vi "CSEI.vi"() -> ()   [LabVIEW 2010]
uses:
  <vilib>/addons/Simulation Interface/_sitctls/sit Indicator Info.ctl
  <vilib>/addons/Simulation Interface/_sitctls/sit Indicator Type.ctl
  <vilib>/addons/Simulation Interface/_sitctls/sit Client Meta Info (v3).ctl
  <vilib>/addons/Simulation Interface/_sitctls/sit MDL Line Item Info.ctl
  <vilib>/addons/Simulation Interface/_sitctls/sit MDL Line Type.ctl
  <vilib>/addons/Simulation Interface/_sitctls/sit Details Settings.ctl
  <vilib>/addons/Simulation Interface/_sitctls/sit Execution Host.ctl
  <vilib>/addons/Simulation Interface/_sitctls/SIT Sim State.ctl
  <vilib>/Utility/inputDevices.llb/closeJoystick.vi
  <vilib>/Utility/inputDevices.llb/joystickAcquire.vi
  <vilib>/addons/Simulation Interface/_sitclient.llb/NI_SIT_sitclient.lvlib
  <vilib>/addons/Simulation Interface/_sitctls/NI_SIT_sitctls.lvlib
  <vilib>/ptbypt/NI_PtbyPt.lvlib
  <vilib>/picture/3D Picture Control/NI_3D Picture Control.lvlib
panel:
  in  "Reset dp":dbl
  in  "eulerselector":dbl=1.0 min=1.0 max=3.0 step=1.0
  in  "xyz selector":dbl=1.0 min=1.0 max=3.0 step=1.0
  out "SIT1 9":dbl
  out "SIT1 8":dbl
  out "SIT1 7":dbl
  out "SIT1 6":dbl
  out "SIT1 5":dbl
  out "SIT1 4":dbl
  out "SIT1 3":dbl
  out "SIT1 2":dbl
  out "SIT1":dbl
  out "stbd vsp r":dbl
  out "port vsp r":dbl
  in  "DPinputFrom":enum32{"OK Button 4", "OK Button 5"}(radio)
  out "SIT_Status":string
  in  "SIT_stopVI":bool
  in  "SIT_Run":bool
  in  "SIT_Pause":bool
  in  "SIT_Stop":bool
  in  "SIT_Details":bool
  in  "SIT_Remap":bool
  in  "SIT_RVE":bool
  in  "CSE1onoff":bool
  in  "Tab Control":T1(tab)
  out "Main battery half voltage":dbl
  out "Servo Battery":dbl(knob) scale=0.0..8.0
  in  "Left Y":dbl(slide) scale=-32676.0..32676.0
  in  "Left X":dbl(slide) scale=-32676.0..32676.0
  out "Bowthruster Battery":dbl(knob) scale=0.0..8.0
  in  "VSP Speeds":dbl(slide) min=-1.0 max=1.0 step=0.05 scale=-1.0..1.0
  out "Main Battery":dbl(knob) scale=0.0..18.0
  in  "Right Y":dbl(slide) scale=-32676.0..32676.0
  in  "Right X":dbl(slide) scale=-32676.0..32676.0
  in  "Power Limiter":dbl(slide) min=0.0 max=1.0 step=0.05 scale=0.0..1.0
  out "Direction L VSP":dbl(knob) scale=180.0..-180.0
  out "Direction R VSP":dbl(knob) scale=180.0..-180.0
  out "Magnitude Pitch L VSP":dbl(knob) scale=0.0..1.0
  out "Magnitude Pitch R VSP":dbl(knob) scale=0.0..1.0
  out "Slide BT green":dbl(slide) scale=0.0..1.0
  out "Slide BT red":dbl(slide)
  out "X button":bool
  out "square":bool
  out "triangle":bool
  out "circle":bool
  out "leftJoystick":bool
  out "rightJoystick":bool
  out "R2button":bool
  out "Dright":bool
  out "Dup":bool
  out "Dleft":bool
  out "Ddown":bool
  out "L2 button":bool
  in  "Eta_d LPF":bool
  in  "Resed DP Int.":bool
  in  "USE cse1 setpoint":bool
  in  "Show HIL":bool
  in  "Show CSEI":bool
  in  "Wave Filter":bool
  in  "K_d":dbl(slide) min=0.0 max=5.0 step=0.25 scale=0.0..5.0
  in  "K_i":dbl(slide) min=0.0 max=5.0 step=0.25 scale=0.0..5.0
  in  "K_p":dbl(slide) min=0.0 max=10.0 step=0.5 scale=0.0..10.0
  out "Vis Yaw":dbl
  out "Vis Pitch":dbl
  out "Vis Roll":dbl
  out "Vis Z":dbl
  out "Vis Y":dbl
  out "Vis X":dbl
  in  "OK Button":bool
  in  "Reset States":dbl
  in  "HIL -> CSE1":bool
  in  "eta_d_Psi":dbl
  in  "eta_d_E":dbl
  in  "eta_d_N":dbl
  out "u5":dbl
  out "u4":dbl
  out "u3":dbl
  out "u2":dbl
  out "u1":dbl
  out "Tau_6":dbl
  out "Tau_2":dbl
  out "Tau_1":dbl
  out "Vis Psi":dbl
  out "Vis E":dbl
  out "Vis N":dbl
  out "3D Picture":refnum<vi>(3d-picture)
  out "Regulation Error Yaw":waveform(dbl)[](graph)
  out "Regulation Error East":waveform(dbl)[](graph)
  out "Regulation Error North":waveform(dbl)[](graph)
  in  "MODE":T2(radio)
  out "Numeric 2":dbl
  out "Numeric":dbl
  in  "Boolean 2":bool
  in  "R2":i32
  in  "L2":i32
  in  "Boolean":bool
  out "Y-axis":i32
  out "X-axis":i32
  out "Joystick Info":T3(array[cluster])
  in  "SIT_Meta_Info":T4
  in  "SIT_Indicator_Indices":T9[](array[typedef])=[{"Indicator Index"=-1, "Number of Signals"=0, "Indicator Type"=enum."Knob"}, {"Indicator Index"=-1, "Number of Signals"=0, "Indicator Type"=enum."Knob"}, {"Indicator Index"=-1, "Number of Signals"=0, "Indicator Type"=enum."Knob"}, {"Indicator Index"=-1, "Number of Signals"=0, "Indicator Type"=enum."Knob"}, {"Indicator Index"=-1, "Number of Signals"=0, "Indicator Type"=enum."Knob"}, {"Indicator Index"=-1, "Number of Signals"=0, "Indicator Type"=enum."Knob"}, {"Indicator Index"=-1, "Number of Signals"=0, "Indicator Type"=enum."Digital"}, {"Indicator Index"=-1, "Number of Signals"=0, "Indicator Type"=enum."Digital"}, {"Indicator Index"=-1, "Number of Signals"=0, "Indicator Type"=enum."Digital"}, {"Indicator Index"=-1, "Number of Signals"=0, "Indicator Type"=enum."WaveformChart"}, {"Indicator Index"=-1, "Number of Signals"=0, "Indicator Type"=enum."WaveformChart"}, {"Indicator Index"=-1, "Number of Signals"=0, "Indicator Type"=enum."WaveformChart"}, {"Indicator Index"=-1, "Number of Signals"=0, "Indicator Type"=enum."Digital"}, {"Indicator Index"=-1, "Number of Signals"=0, "Indicator Type"=enum."Digital"}, {"Indicator Index"=-1, "Number of Signals"=0, "Indicator Type"=enum."Digital"}, {"Indicator Index"=-1, "Number of Signals"=0, "Indicator Type"=enum."Digital"}, {"Indicator Index"=-1, "Number of Signals"=0, "Indicator Type"=enum."Digital"}, {"Indicator Index"=-1, "Number of Signals"=0, "Indicator Type"=enum."Digital"}, {"Indicator Index"=-1, "Number of Signals"=0, "Indicator Type"=enum."Digital"}, {"Indicator Index"=-1, "Number of Signals"=0, "Indicator Type"=enum."Digital"}, {"Indicator Index"=-1, "Number of Signals"=0, "Indicator Type"=enum."Digital"}, {"Indicator Index"=-1, "Number of Signals"=0, "Indicator Type"=enum."Knob"}, {"Indicator Index"=-1, "Number of Signals"=0, "Indicator Type"=enum."Slide"}, {"Indicator Index"=-1, "Number of Signals"=0, "Indicator Type"=enum."Slide"}, {"Indicator Index"=-1, "Number of Signals"=0, "Indicator Type"=enum."Digital"}, {"Indicator Index"=-1, "Number of Signals"=0, "Indicator Type"=enum."Digital"}, {"Indicator Index"=-1, "Number of Signals"=0, "Indicator Type"=enum."Digital"}, {"Indicator Index"=27, "Number of Signals"=1, "Indicator Type"=enum."Digital"}, {"Indicator Index"=28, "Number of Signals"=1, "Indicator Type"=enum."Digital"}, {"Indicator Index"=-1, "Number of Signals"=0, "Indicator Type"=enum."Digital"}, {"Indicator Index"=30, "Number of Signals"=1, "Indicator Type"=enum."Digital"}, {"Indicator Index"=-1, "Number of Signals"=0, "Indicator Type"=enum."Digital"}, {"Indicator Index"=-1, "Number of Signals"=0, "Indicator Type"=enum."Digital"}, {"Indicator Index"=-1, "Number of Signals"=0, "Indicator Type"=enum."Digital"}, {"Indicator Index"=-1, "Number of Signals"=0, "Indicator Type"=enum."Digital"}, {"Indicator Index"=-1, "Number of Signals"=0, "Indicator Type"=enum."Digital"}, {"Indicator Index"=-1, "Number of Signals"=0, "Indicator Type"=enum."Boolean"}, {"Indicator Index"=-1, "Number of Signals"=0, "Indicator Type"=enum."Digital"}, {"Indicator Index"=-1, "Number of Signals"=0, "Indicator Type"=enum."Digital"}, {"Indicator Index"=-1, "Number of Signals"=0, "Indicator Type"=enum."Digital"}, {"Indicator Index"=-1, "Number of Signals"=0, "Indicator Type"=enum."Digital"}, {"Indicator Index"=-1, "Number of Signals"=0, "Indicator Type"=enum."Digital"}, {"Indicator Index"=-1, "Number of Signals"=0, "Indicator Type"=enum."Digital"}, {"Indicator Index"=-1, "Number of Signals"=0, "Indicator Type"=enum."Digital"}]
  # "MODE"
  # "TARGET"
  # "DP Controller Input Selector"
  # "Model Controls"
  # "CS Enterprise I"
  # "HID Info"
  # "Workaround for Qualisys probllems!!!"
  # "Voltages"
  # "Actuators"
  # "SONY Dualshock3 SIXAXIS"
  # "Port Tunnel Thruster (L2)\n(Negative Yaw Moment)"
  # "Starboard Tunnel Thruster (R2)\n(Positive Yaw Moment)"
  # "Bowthruster"
  # "Increase BT power limit"
  # "VSP Speeds"
  # "Increase VSP speed"
  # "Decrease BT power limit"
  # "Starboard full CCW\nPort full CW"
  # "Starboard full CW\nPort full CCW"
  # "Decrease VSP speed"
  # "VSP pitch"
  # "Bow Thruster Power Limit"
  # "Starboard VSP"
  # "Port VSP\n(surge/sway force setpoint)"
  # "PS3 joysticks"
  # "DP Setpoints"
  # "Misc"
  # "DP controller gains"
  # "HIL"
  # "Toggle visibility"
  # "CS Enterprise I"
  # "Toggle visibility"
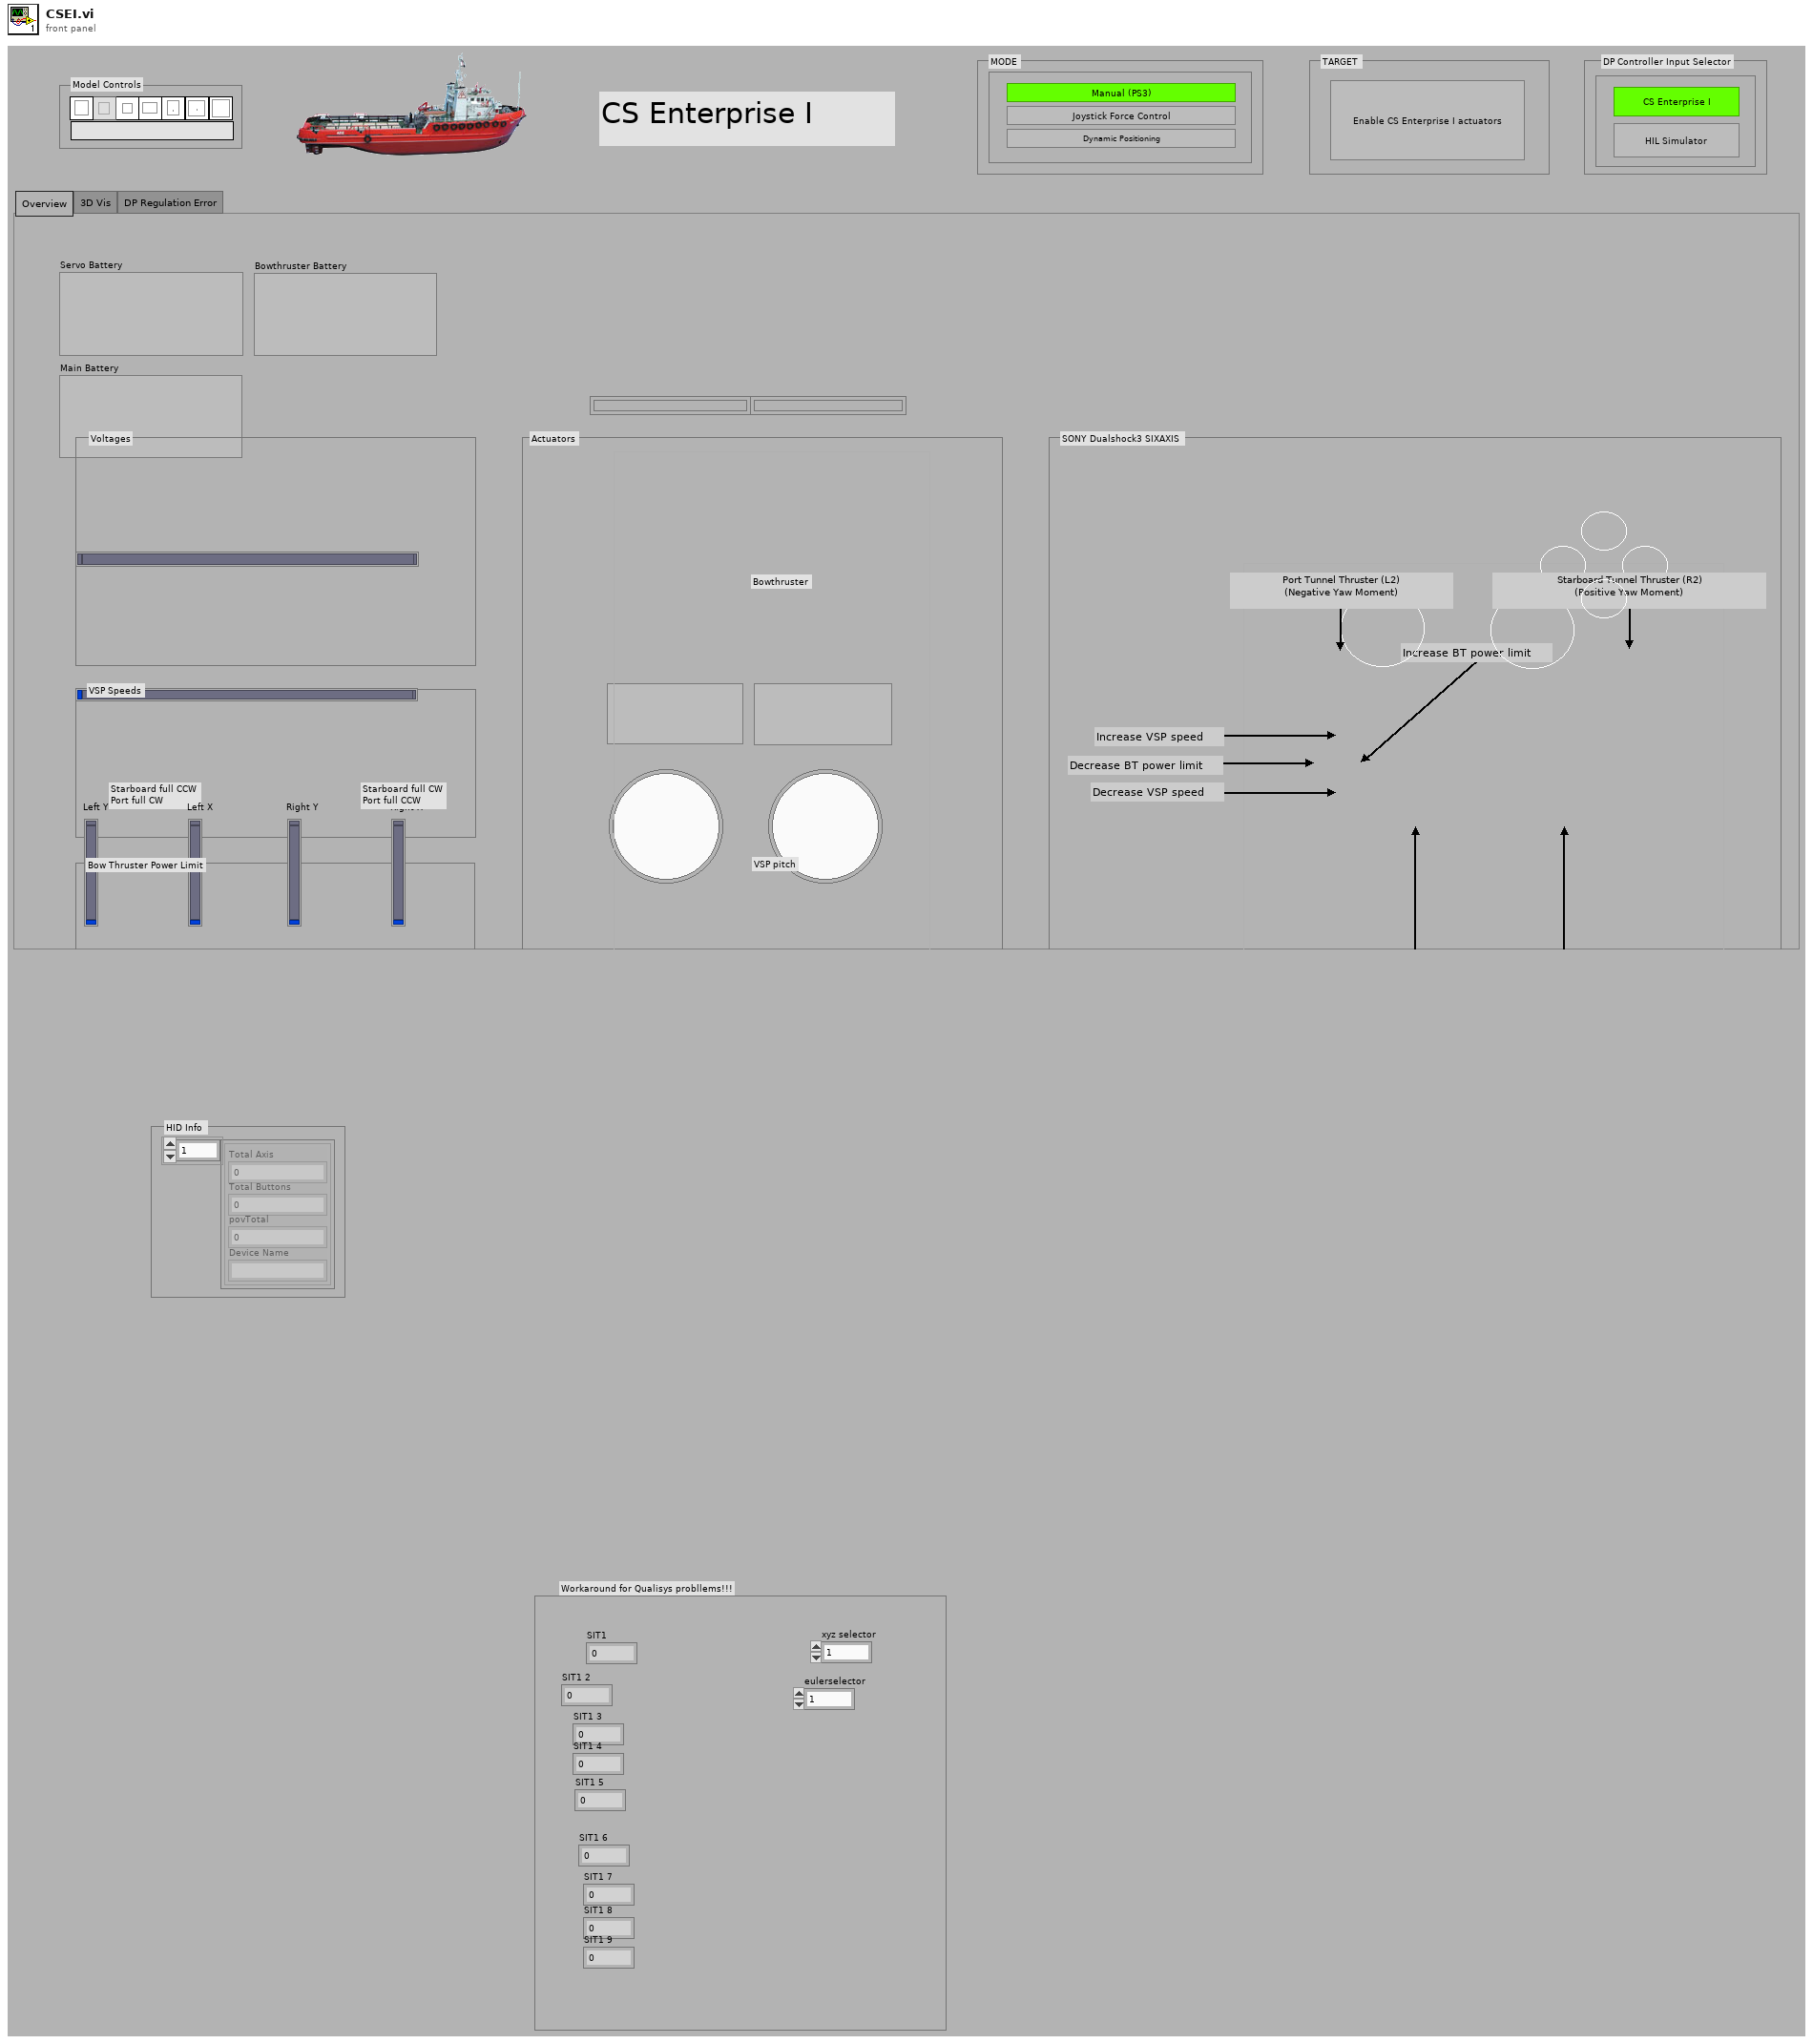
[diagram p1: front panel]
types:
  T1 = enum32{"Overview", "3D Vis", "DP Regulation Error"}
  T2 = enum32{"OK Button 4", "OK Button 5", "OK Button 6"}
  T3 = cluster{"Total Axis":u32, "Total Buttons":u32, "povTotal":u32, "Device Name":string}[]
  T4 = typedef "NI_SIT_sitctls.lvlib/sit Client Meta Info (v3).ctl" = cluster{"Simulation IP":string, "Target IP":string, "Host Port":u16, "Model DLL Path":path, "Model File Path":path, "Model Name":string, "Param Tree Info ":T5[], "Signal Tree Info":T5[], "Details Settings":T7, "Client Name":string, "Stored Model Checksum":string, "Buffer Sizes":cluster{"number of signals":u32, "circular buffer size":u32, "num data points":u32}, "Execution Host":T8, "Project Dir":path, "Last MDL":path}
  T5 = typedef "NI_SIT_sitctls.lvlib/sit MDL Line Item Info.ctl" = cluster{"Line Type":T6, "Section Type":string, "Name":string, "Value":string, "Owner Index":i32, "Tree Tag":string, "Child Indices":i32[], "Expanded?":bool, "Destination Block Info":string[]}
  T6 = typedef "NI_SIT_sitctls.lvlib/sit MDL Line Type.ctl" = enum16{"Section Head", "Parameter", "Section End", "Comment"}
  T7 = typedef "NI_SIT_sitctls.lvlib/sit Details Settings.ctl" = cluster{"Halt on Task Overrun?":bool, "Halt on Lost Data?":bool, "Signal Decimation":i32, "Autoscale":bool}
  T8 = typedef "NI_SIT_sitctls.lvlib/sit Execution Host.ctl" = enum32{"Simulation Environment", "RT Target", "Local Driver"}
  T9 = typedef "NI_SIT_sitctls.lvlib/sit Indicator Info.ctl" = cluster{"Indicator Index":i32, "Number of Signals":i32, "Indicator Type":T10}
  T10 = typedef "NI_SIT_sitctls.lvlib/sit Indicator Type.ctl" = enum32{"xxx1", "xxx2", "xxx3", "Generic   ", "Decoration", "Text", "xControl", "ColorBox", "Boolean", "RefNum", "Variant", "Path", "ListBox", "Table", "Array", "Picture", "ActiveXContainer", "Numeric", "Digital", "NamedNumeric", "ColorRamp", "Slide", "GraphOrChart", "WaveformChart", "WaveformGraph", "IntensityChart", "xxx4", "xxx5", "xxx6", "xxx7", "Cluster", "Panel", "Knob", "NumWithScale", "Ring", "Enum", "GObject", "Plot", "Cursor", "NumericText", "Scale", "ColorScale", "GraphScale", "ColorGraphScale", "TypedRefNum", "OldKnobScale", "MCListbox", "WaveformData", "BVTag", "DAQName", "VISAName", "IVIName", "SlideScale"}
  T11 = cluster{"Red":sgl, "Green":sgl, "Blue":sgl, "Alpha":sgl}
  T12 = cluster{"axes total":u32, "buttons total":u32, "pov total":u32, "device name":string}[]
  T13 = cluster{"X axis":i32, "Y axis":i32, "Z axis":i32, "X axis rotation":i32, "Y axis rotation":i32, "Z axis rotation":i32, "U axis":i32, "V axis":i32}
  T14 = cluster{"button 1":bool, "button 2":bool, "button 3":bool, "button 4":bool, "button 5":bool, "button 6":bool, "button 7":bool, "button 8":bool, "button 9":bool, "button 10":bool, "button 11":bool, "button 12":bool, "button 13":bool, "button 14":bool, "button 15":bool, "button 16":bool, "button 17":bool, "button 18":bool, "button 19":bool, "button 20":bool, "button 21":bool, "button 22":bool, "button 23":bool, "button 24":bool, "button 25":bool, "button 26":bool, "button 27":bool, "button 28":bool, "button 29":bool, "button 30":bool, "button 31":bool, "button 32":bool}
  T15 = cluster{"pov 1":i32, "pov 2":i32, "pov 3":i32, "pov 4":i32}
  T16 = typedef "NI_SIT_sitctls.lvlib/sit TCP Conn and Queue.ctl" = cluster{"TCP Connection":refnum<k5>, "Data Queue":refnum<queue>, "Execution Host":T8}
  T17 = typedef "NI_SIT_sitctls.lvlib/sit Client Op Refs.ctl" = cluster{"Conn and Queue":T16, "RunPauseStop Refs":refnum<vi>[], "Control Refs":refnum<vi>[], "Indicator Refs":refnum<vi>[], "Param Info":T18[], "State Queue":refnum<queue>, "Don't Modify Scales?":bool, "Param Info Needs Init?":bool}
  T18 = typedef "NI_SIT_sitctls.lvlib/SIT param info.ctl" = cluster{"paramidx":i32, "ID":string, "paramname":string, "dattype":i32, "Dimensions":i32[], "value":dbl[]}
  T19 = typedef "NI_SIT_sitctls.lvlib/SIT Sim State.ctl" = enum8{"Default", "Idle", "Running", "Paused", "Stopped", "Error"}
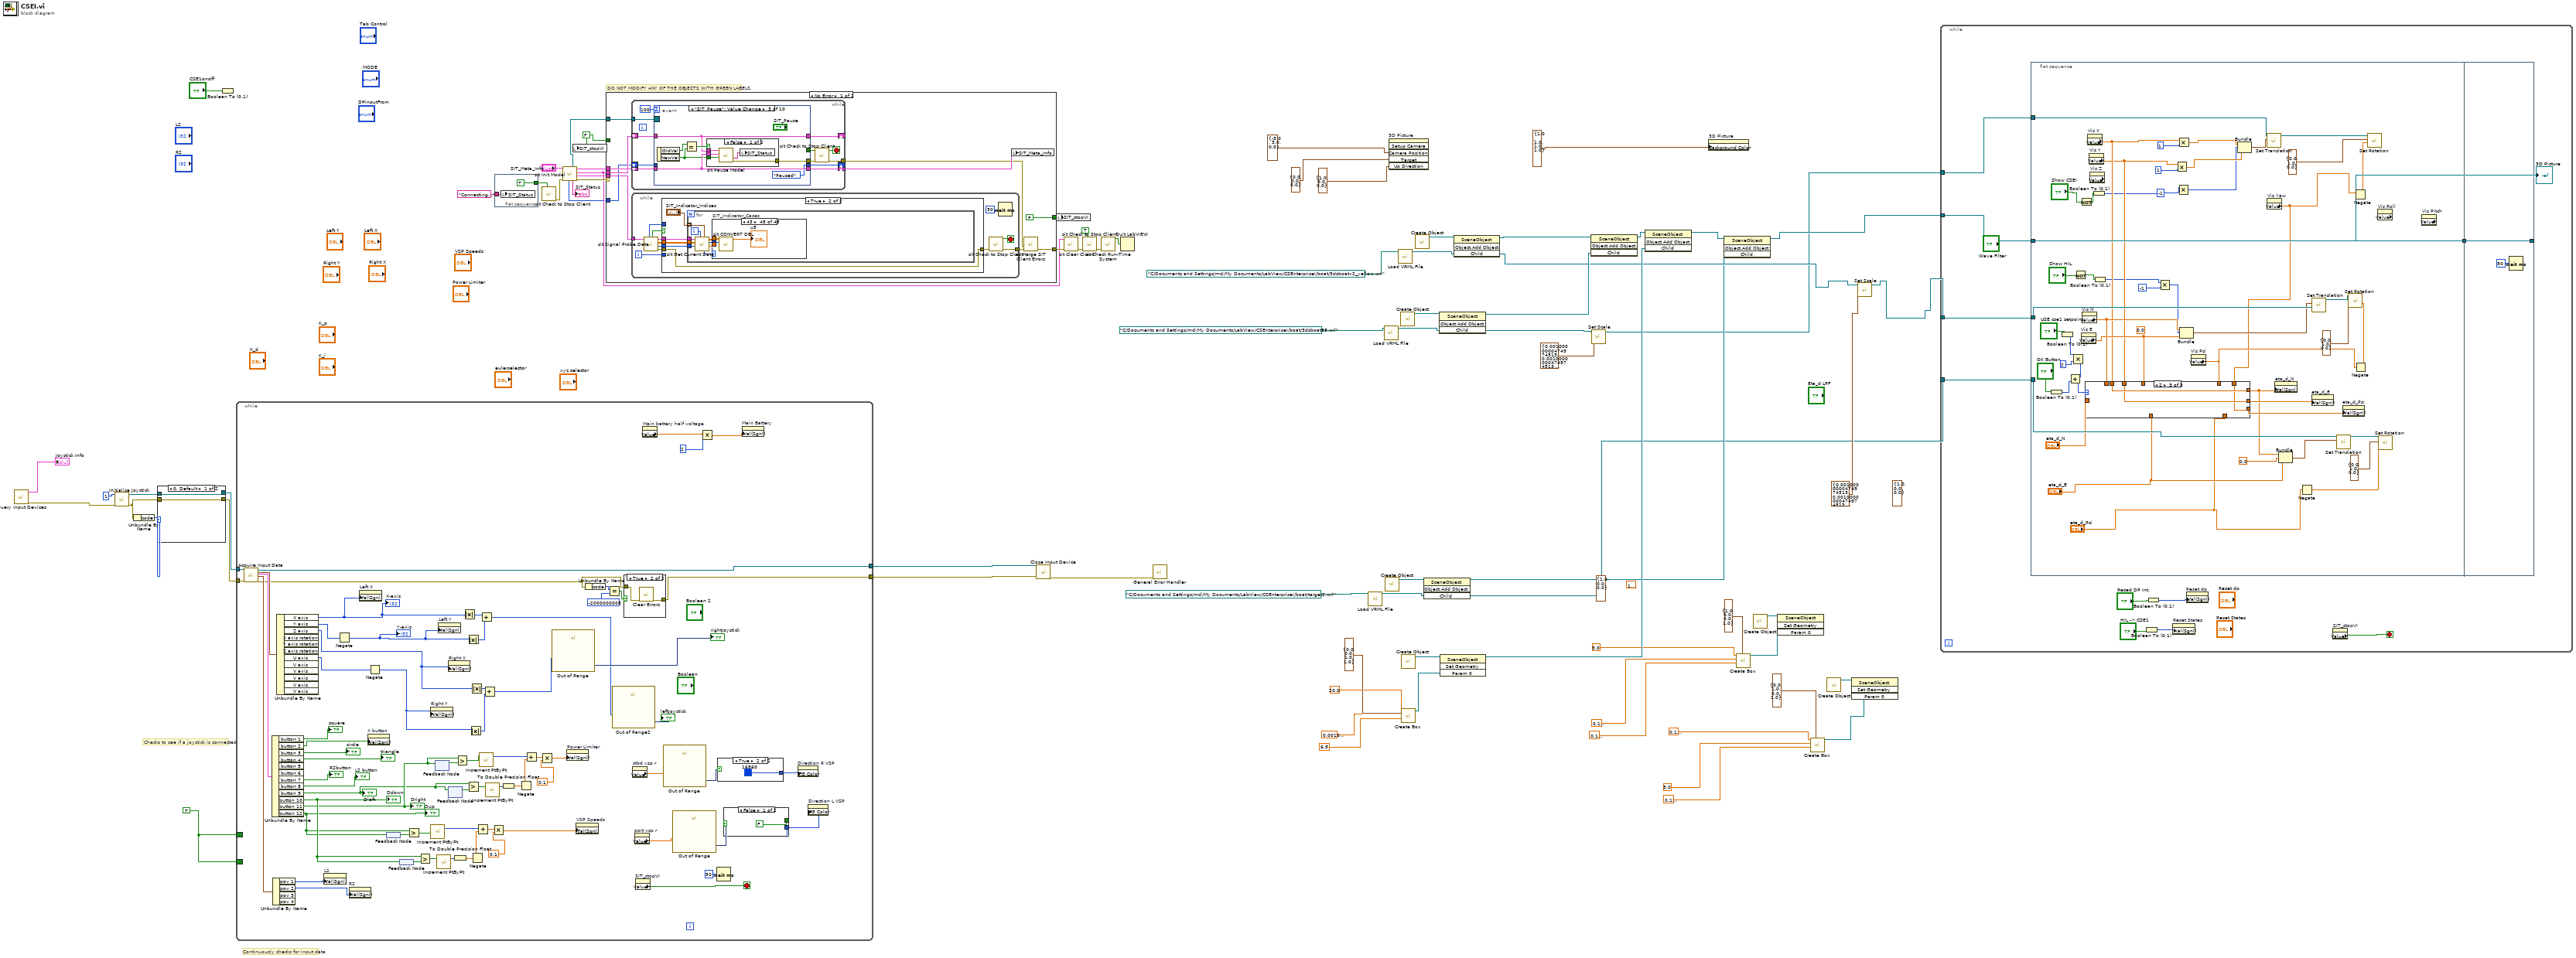
[diagram p0: block diagram]
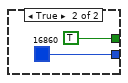
[diagram p6: hidden frame]
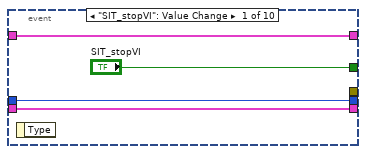
[diagram p8: hidden frame]
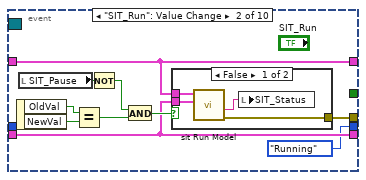
[diagram p9: hidden frame]
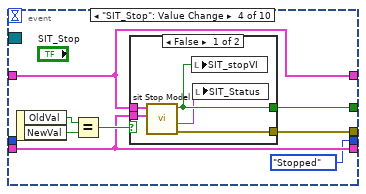
[diagram p12: hidden frame]
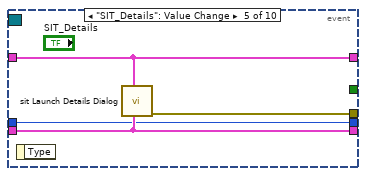
[diagram p14: hidden frame]
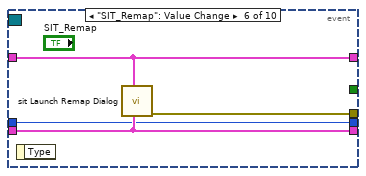
[diagram p15: hidden frame]
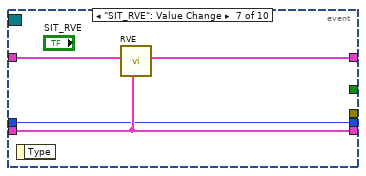
[diagram p16: hidden frame]
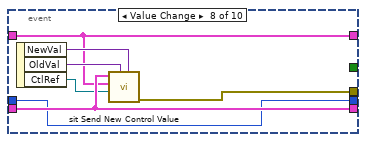
[diagram p17: hidden frame]
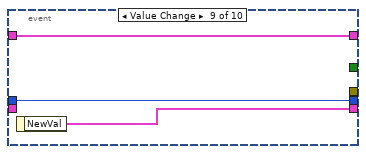
[diagram p18: hidden frame]
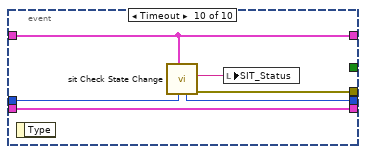
[diagram p19: hidden frame]
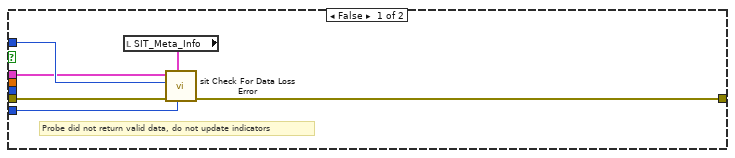
[diagram p20: hidden frame]
diagram:
  (unwired) cluster{"X":sgl, "Y":sgl, "Z":sgl} {"X"=1.0, "Y"=0.0, "Z"=0.0} ("Camera Position")
  (unwired) 1.5707963267948966
  (unwired) cluster{"X":sgl, "Y":sgl, "Z":sgl} {"X"=1.0, "Y"=0.0, "Z"=0.0} ("Camera Position")
  w47 = TRUE
  w66 = FALSE
  # "Continuously checks for input data"
  # "Checks to see if a joystick is connected"
  # "DO NOT MODIFY ANY OF THE OBJECTS WITH GREEN LABELS."
  n1 = call <vilib>:"Query Input Devices.vi"() -> ("error out"=w58:errorcluster, "joystick info"=→"Joystick Info":T12)  [unwired: 1 in, 9 out]
  n2 = call <vilib>:"Initialize Joystick.vi"("error in (no error)"=w58, "device index"=1) -> ("error out"=w51:errorcluster, "device ID"=w52:refnum<k1>)  [unwired: 8 out]
  n3 = Unbundle By Name(w51) -> ("code"=w53:i32)
  n4 = case shown="0, Default" w53 {
    tunnel: w51 -> [w78 w80]
    tunnel: [w78 w80] -> w50
    tunnel: w52 -> [w77 w79]
    tunnel: [w77 w79] -> w49
    frame 0, Default {
    }
    frame -2000000008 {
    }
  }
  n5 = Boolean To (0,1)(Boolean="CSE1onoff") -> ()  [unwired: 1 out]
  n6 = while {
    tunnel: [w142] -> w55
    tunnel: [w146] -> w56
    tunnel: w50 -> [w140]
    tunnel: w49 -> [w139]
    border: w47 -> [_]
    border: w47 -> [_]
    stop <- w138 stop-if-true
    n7 = call-poly <vilib>:"Acquire Input Data.vi"("device ID"=w139, "error in (no error)"=w140) -> ("device ID"=w146:refnum<k1>, "axis info"=w150:T13, "button info"=w149:T14, "direction info"=w148:T15, "error out"=w141:errorcluster)  [unwired: 13 out]
    n8 = Unbundle By Name(w149) -> ("button 1"=→"square":bool, "button 2"=w90:bool, "button 3"=→"circle":bool, "button 4"=→"triangle":bool, "button 7"=→"R2button":bool, "button 8"=→"L2 button":bool, "button 9"=w104:bool, "button 10"=w117:bool, "button 11"=w105:bool, "button 12"=w116:bool)  [unwired: 2 out]
    "Dleft" <- w104
    "Ddown" <- w117
    "Dup" <- w116
    "Dright" <- w105
    n9 = Unbundle By Name(w148) -> ("pov 1"=w102:i32, "pov 2"=w101:i32)  [unwired: 2 out]
    n10 = Unbundle By Name(w150) -> ("X axis"=w87:i32, "Y axis"=w136:i32, "Z axis"=w85:i32, "U axis"=w137:i32)  [unwired: 8 out]
    "X-axis" <- w87
    n11 = property on="L2" class="DigNum (strict)"("Val(Sgnl)"=w102) -> ()  [unwired: 2 in, 2 out]
    n12 = Negate(x=w136) -> (-x=w86:i32)
    "Y-axis" <- w86
    n13 = property on="R2" class="DigNum (strict)"("Val(Sgnl)"=w101) -> ()  [unwired: 2 in, 2 out]
    n14 = property on="Left X" class="Slide (strict)"("Val(Sgnl)"=w87) -> ()  [unwired: 2 in, 2 out]
    n15 = property on="X button" class="Bool (strict)"("Val(Sgnl)"=w90) -> ()  [unwired: 2 in, 2 out]
    n16 = Negate(x=w137) -> (-x=w84:i32)
    n17 = feedback-in #1(w116) -> ()
    n18 = feedback #1() -> (w135:bool)
    n19 = feedback #2() -> (w133:bool)
    n20 = feedback-in #2(w117) -> ()
    n21 = Greater?(x=w116, y=w135) -> (0:w134:bool)
    n22 = Greater?(x=w117, y=w133) -> (0:w132:bool)
    n23 = property on="Right Y" class="Slide (strict)"("Val(Sgnl)"=w84) -> ()  [unwired: 2 in, 2 out]
    n24 = call <vilib>:"Increment PtByPt.vi"("activate"=w134) -> ("counter"=w131:u32)  [unwired: 1 in, 1 out]
    n25 = feedback #3() -> (w115:bool)  [unwired: 1 in]
    n26 = feedback-in #3(w105) -> ()
    n27 = call <vilib>:"Increment PtByPt.vi"("activate"=w132) -> ("counter"=w129:u32)  [unwired: 1 in, 1 out]
    n28 = property on="Left Y" class="Slide (strict)"("Val(Sgnl)"=w86) -> ()  [unwired: 2 in, 2 out]
    n29 = property on="Right X" class="Slide (strict)"("Val(Sgnl)"=w85) -> ()  [unwired: 2 in, 2 out]
    n30 = feedback #4() -> (w113:bool)  [unwired: 1 in]
    n31 = feedback-in #4(w104) -> ()
    n32 = To Double Precision Float(number=w129) -> (double precision float=w128:dbl)
    n33 = Greater?(x=w105, y=w115) -> (0:w114:bool)
    n34 = Absolute Value(x=w87) -> (abs(x)=w122:i32)
    n35 = Absolute Value(x=w86) -> (abs(x)=w121:i32)
    n36 = Greater?(x=w104, y=w113) -> (0:w112:bool)
    n37 = Absolute Value(x=w84) -> (abs(x)=w119:i32)
    n38 = Absolute Value(x=w85) -> (abs(x)=w120:i32)
    n39 = Negate(x=w128) -> (-x=w130:dbl)
    n40 = Add(x=w131, y=w130) -> (x+y=w127:dbl)
    n41 = call <vilib>:"Increment PtByPt.vi"("activate"=w114) -> ("counter"=w111:u32)  [unwired: 1 in, 1 out]
    n42 = Add(x=w122, y=w121) -> (x+y=w97:i32)
    n43 = Add(x=w120, y=w119) -> (x+y=w96:i32)
    n44 = call <vilib>:"Increment PtByPt.vi"("activate"=w112) -> ("counter"=w109:u32)  [unwired: 1 in, 1 out]
    n45 = Multiply(x=w127, y=0.1) -> (x*y=w89:dbl)
    n46 = To Double Precision Float(number=w109) -> (double precision float=w108:dbl)
    n47 = Negate(x=w108) -> (-x=w110:dbl)
    n48 = Add(x=w111, y=w110) -> (x+y=w107:dbl)
    n49 = Multiply(x=w107, y=0.1) -> (x*y=w103:dbl)
    n50 = call "Out of Range"("Operand 1"=w96) -> ("Result"=→"rightJoystick":dynamicdata)  [unwired: 9 in, 1 out]
    n51 = property on="Power Limiter" class="Slide (strict)"("Val(Sgnl)"=w103) -> ()  [unwired: 2 in, 2 out]
    n52 = property on="VSP Speeds" class="Slide (strict)"("Val(Sgnl)"=w89) -> ()  [unwired: 2 in, 2 out]
    n53 = Unbundle By Name(w141) -> ("code"=w145:i32)
    n54 = Equal?(x=w145, y=-2000000008) -> (x = y?=w143:bool)
    n55 = call "Out of Range2"("Operand 1"=w97) -> ("Result"=→"leftJoystick":dynamicdata)  [unwired: 9 in, 1 out]
    n56 = case shown="True" w143 {
      tunnel: w141 -> [w157 w159]
      tunnel: [w157 w158] -> w142
      frame False {
      }
      frame True {
        n57 = call <vilib>:"Clear Errors.vi"("error in (no error)"=w159) -> ("error out"=w158:errorcluster)  [unwired: 6 out]
      }
    }
    n58 = property on="stbd vsp r" class="DigNum (strict)"() -> ("Value"=w91:dbl)  [unwired: 2 in, 2 out]
    n59 = property on="port vsp r" class="DigNum (strict)"() -> ("Value"=w92:dbl)  [unwired: 2 in, 2 out]
    n60 = property on="SIT_stopVI" class="Bool (strict)"() -> ("Value"=w138:bool)  [unwired: 2 in, 2 out]
    n61 = property on="Main battery half voltage" class="DigNum (strict)"() -> ("Value"=w83:dbl)  [unwired: 2 in, 2 out]
    n62 = call "Out of Range"("Operand 1"=w91) -> ("Result"=w95:dynamicdata)  [unwired: 9 in, 1 out]
    n63 = call "Out of Range"("Operand 1"=w92) -> ("Result"=w93:dynamicdata)  [unwired: 9 in, 1 out]
    n64 = Multiply(x=w83, y=2) -> (x*y=w82:dbl)
    n65 = Wait (ms)(milliseconds to wait=u32 50) -> ()  [unwired: 1 out]
    n66 = case shown="True" w95 {
      tunnel: [u32 16777216 u32 16860] -> w118
      frame False {
      }
      frame True {
      }
    }
    n67 = case shown="False" w93 {
      tunnel: [u32 16777216 u32 16860] -> w125
      tunnel: [FALSE TRUE] -> _
      frame False {
      }
      frame True {
      }
    }
    n68 = property on="Main Battery" class="Knob (strict)"("Val(Sgnl)"=w82) -> ()  [unwired: 2 in, 2 out]
    n69 = property on="Direction R VSP" class="Knob (strict)"("FG Color"=w118) -> ()  [unwired: 2 in, 2 out]
    n70 = property on="Direction L VSP" class="Knob (strict)"("FG Color"=w125) -> ()  [unwired: 2 in, 2 out]
  }
  n71 = flat-sequence {
    tunnel: [TRUE ("Clear Item?")] -> w70
    tunnel: "Connecting..." ("SIT_Status") -> [w160]
    frame #0 {
      n72 = local write "SIT_Status"(w160) -> ()
    }
  }
  n73 = call <vilib>:"sit Check to Stop Client.vi"("Reset Stop?"=w70) -> ("error out"=w72:errorcluster)  [unwired: 2 in, 8 out]
  n74 = call <vilib>:"sit Init Model.vi"("error in (no error)"=w72, "SIT_Meta_Info in"="SIT_Meta_Info") -> ("error out"=w76:errorcluster, "Conn and Queue"=w63:T16, "SIT Client Op Refs"=w67:T17, "SIT_Meta_Info out"=w74:T4, "Initial State"=→"SIT_Status":string, "Event Registration Refnum"=w75:refnum<event-registration>, "State"=w64:T19)  [unwired: 2 in, 1 out]
  n75 = local write "SIT_stopVI"(w66) -> ()
  n76 = case shown="No Error" w76 {
    selector: w76 -> [_ w426]
    tunnel: w75 -> [w171 _]
    tunnel: w74 -> [w169 w425]
    tunnel: [w165 w426] -> w71
    tunnel: w67 -> [w168 _]
    tunnel: w66 -> [_ _]
    tunnel: [FALSE _] -> w65
    tunnel: w64 -> [w163 _]
    tunnel: w63 -> [w162 _]
    frame No Error {
      n77 = while {
        tunnel: w171 -> [w183]
        tunnel: [w181] -> w164
        shift-right: [w175] -> _
        shift-left: w168 -> [w179]
        shift-right: [w182] -> w170
        shift-left: w169 -> [w180]
        shift-right: [w172] -> _
        shift-left: w163 -> [w173]
        stop <- w174 stop-if-true
        n78 = event shown="[2] \"SIT_Pause\": Value Change" {
          selector: w183 -> [_ _ _ _ _ _ _ _ _ _]
          dyn-events: _ -> [_ _ _ _ _ _ _ _ _ _]
          timeout: 100 -> [_ _ _ _ _ _ _ _ _ _]
          tunnel: ["SIT_stopVI" _ _ w218 _ _ _ _ _ _] -> w176
          tunnel: [_ w193 w205 w217 w230 w234 _ w245 _ w252] -> w177
          tunnel: w180 -> [w186 w191 w206 w219 w229 w233 w237 w244 _ w254]
          tunnel: w179 -> [w184 w192 w207 w220 w228 w231 w238 w240 w247 w253]
          tunnel: [w186 w191 w206 w219 w229 w233 w237 w244 w248 w254] -> w182
          tunnel: [w184 w192 w207 w220 w228 w231 w236 w240 w247 w253] -> w175
          tunnel: [w185 SIT_Sim_State."Running" ("State") SIT_Sim_State."Paused" ("State") SIT_Sim_State."Stopped" ("State") w227 w232 w235 w239 w246 w250] -> w172
          tunnel: w173 -> [w185 _ _ _ w227 w232 w235 w239 w246 w251]
          event "SIT_stopVI": Value Change {
            n79 = event-data() -> ()  [unwired: 2 out]
          }
          event "SIT_Run": Value Change {
            n80 = event-data() -> ("OldVal"=w189:bool, "NewVal"=w190:bool)  [unwired: 1 out]
            n81 = local read "SIT_Pause"() -> (w196:bool)
            n82 = Equal?(x=w189, y=w190) -> (x = y?=w194:bool)
            n83 = Not(x=w196) -> (.not. x?=w197:bool)
            n84 = And(x=w197, y=w194) -> (x .and. y?=w195:bool)
            n85 = case shown="False" w195 {
              tunnel: [w201 _] -> w193
              tunnel: w192 -> [w200 _]
              tunnel: w191 -> [w199 _]
              frame False {
                n86 = call <vilib>:"sit Run Model.vi"("SIT Meta Info"=w199, "SIT Client Op Refs"=w200) -> ("error out"=w201:errorcluster, "Status"=w198:string)  [unwired: 6 in, 2 out]
                n87 = local write "SIT_Status"(w198) -> ()
              }
              frame True {
                # "Ignore value change if it is\nto the same value"
              }
            }
          }
          event "SIT_Pause": Value Change {
            n88 = event-data() -> ("OldVal"=w203:bool, "NewVal"=w204:bool)  [unwired: 1 out]
            n89 = Equal?(x=w203, y=w204) -> (x = y?=w208:bool)
            n90 = case shown="False" w208 {
              tunnel: [w213 _] -> w205
              tunnel: w207 -> [w212 _]
              tunnel: w206 -> [w211 _]
              tunnel: w204 -> [w210 _]
              frame False {
                n91 = call <vilib>:"sit Pause Model.vi"("Pause Button Value"=w210, "SIT Meta Info"=w211, "SIT Client Op Refs"=w212) -> ("error out"=w213:errorcluster, "Status"=w209:string)  [unwired: 3 in, 4 out]
                n92 = local write "SIT_Status"(w209) -> ()
              }
              frame True {
                # "Ignore value change if it is\nto the same value"
              }
            }
          }
          event "SIT_Stop": Value Change {
            n93 = event-data() -> ("OldVal"=w215:bool, "NewVal"=w216:bool)  [unwired: 1 out]
            n94 = Equal?(x=w215, y=w216) -> (x = y?=w221:bool)
            n95 = case shown="False" w221 {
              tunnel: [w226 _] -> w217
              tunnel: [w223 _] -> w218
              tunnel: w219 -> [w225 _]
              tunnel: w220 -> [w224 _]
              frame False {
                n96 = call <vilib>:"sit Stop Model.vi"("SIT Meta Info"=w225, "SIT Client Op Refs"=w224) -> ("error out"=w226:errorcluster, "Status"=w222:string, "Stop VI?"=w223:bool)  [unwired: 4 in, 3 out]
                n97 = local write "SIT_stopVI"(w223) -> ()
                n98 = local write "SIT_Status"(w222) -> ()
              }
              frame True {
                # "Ignore value change if it is\nto the same value"
              }
            }
          }
          event "SIT_Details": Value Change {
            n99 = event-data() -> ()  [unwired: 2 out]
            n100 = call <vilib>:"sit Launch Details Dialog.vi"("SIT Meta Info in"=w229, "SIT Client Op Refs"=w228) -> ("error out"=w230:errorcluster)  [unwired: 1 in, 8 out]
          }
          event "SIT_Remap": Value Change {
            n101 = event-data() -> ()  [unwired: 2 out]
            n102 = call <vilib>:"sit Launch Remap Dialog.vi"("SIT Meta Info in"=w233, "SIT Client Op Refs"=w231) -> ("error out"=w234:errorcluster)  [unwired: 2 in, 7 out]
          }
          event "SIT_RVE": Value Change {
            n103 = event-data() -> ()  [unwired: 2 out]
            n104 = call <vilib>:"RVE.vi"("SIT_Meta_Info"=w237, "SIT Client Op Refs in"=w238) -> ("SIT Client Op Refs out"=w236:T17)  [unwired: 9 out]
          }
          event Value Change {
            n105 = event-data() -> ("NewVal"=w241:variant, "OldVal"=w242:variant, "CtlRef"=w243:refnum<vi>)  [unwired: 1 out]
            n106 = call <vilib>:"sit Send New Control Value.vi"("Control New Value"=w241, "Control Old Value"=w242, "Control Ref"=w243, "SIT Client Op Refs"=w240, "SIT_Meta_Info"=w244) -> ("error out"=w245:errorcluster)  [unwired: 4 in, 2 out]
          }
          event Value Change {
            n107 = event-data() -> ("NewVal"=w248:T4)  [unwired: 1 out]
          }
          event Timeout {
            n108 = event-data() -> ()  [unwired: 2 out]
            n109 = call <vilib>:"sit Check State Change.vi"("Old State in"=w251, "SIT Client Op Refs"=w253) -> ("error out"=w252:errorcluster, "Status String"=w249:string, "New State out"=w250:T19)  [unwired: 7 out]
            n110 = local write "SIT_Status"(w249) -> ()
          }
        }
        n111 = call <vilib>:"sit Check to Stop Client.vi"("error in (no error)"=w177, "User Stop?"=w176) -> ("error out"=w181:errorcluster, "Stop?"=w174:bool)  [unwired: 1 in, 7 out]
      }
      n112 = while "Read Loop" {
        tunnel: [w265] -> w166
        tunnel: w162 -> [w255]
        i -> [w262]
        stop <- w263 stop-if-true
        n113 = call <vilib>:"sit Signal Probe Data.vi"("TCP Conn and Queue"=w255) -> ("error out"=w258:errorcluster, "Dimensions"=w259:i32[], "Raw Data"=w260:dbl[][], "dup TCP Conn and Queue"=w261:T16, "Valid Data?"=w256:bool, "Options out"=w257:u32)  [unwired: 4 in, 1 out]
        n114 = case shown="True" w256 {
          tunnel: w260 -> [_ w276]
          tunnel: w259 -> [_ w275]
          tunnel: w261 -> [w268 w274]
          tunnel: w258 -> [w271 w273]
          tunnel: [w270 w273] -> w264
          tunnel: w257 -> [w272 _]
          tunnel: w262 -> [w269 _]
          frame False {
            # "Probe did not return valid data, do not update indicators"
            n115 = local read "SIT_Meta_Info"() -> (w267:T4)
            n116 = call <vilib>:"sit Check For Data Loss Error.vi"("Iteration"=w269, "SIT Meta Info"=w267, "error in (no error)"=w271, "Options"=w272, "TCP Conn and Queue"=w268) -> ("error out"=w270:errorcluster)  [unwired: 6 out]
          }
          frame True {
            n117 = for {
              tunnel: w276 -> [w286]
              tunnel: "SIT_Indicator_Indices" -> [w282] mode=indexing
              tunnel: w275 -> [w285]
              tunnel: w274 -> [w283]
              i -> [w284]
              n118 = call <vilib>:"sit Get Current Data.vi"("Indicator Index Cluster"=w282, "Iteration"=w284, "Dimensions"=w285, "Raw Data"=w286, "Conn and Queue"=w283) -> ("Timestamps"=w279:dbl[], "Last Row"=w280:i32, "Current Data"=w281:dbl[][], "Indicator Index"=w278:i32)  [unwired: 1 in, 2 out]
              n119 = case "SIT_Indicator_Cases" shown="43" w278 {
                tunnel: w281 -> [_ w289 w292 w295 w298 w301 w304 w307 w310 w313 w317 w322 w327 w331 w334 w337 w340 w343 w346 w349 w352 w355 w358 w361 w364 w367 w370 w373 w376 w379 w382 w385 w388 w391 w394 w397 w400 w403 w406 w409 w412 w415 w418 w421 w424]
                tunnel: w280 -> [_ w288 w291 w294 w297 w300 w303 w306 w309 w312 w316 w321 w326 w330 w333 w336 w339 w342 w345 w348 w351 w354 w357 w360 w363 w366 w369 w372 w375 w378 w381 w384 w387 w390 w393 w396 w399 w402 w405 w408 w411 w414 w417 w420 w423]
                tunnel: w279 -> [_ _ _ _ _ _ _ _ _ _ w315 w320 w325 _ _ _ _ _ _ _ _ _ _ _ _ _ _ _ _ _ _ _ _ _ _ _ _ _ _ _ _ _ _ _ _]
                frame -1, Default {
                }
                frame 0 {
                  n120 = call <vilib>:"sit CONVERT DBL.vi"("Last Row"=w288, "Raw Data"=w289) -> ("Output"=→"Bowthruster Battery":dbl)  [unwired: 9 in]
                }
                frame 1 {
                  n121 = call <vilib>:"sit CONVERT DBL.vi"("Last Row"=w291, "Raw Data"=w292) -> ("Output"=→"Direction L VSP":dbl)  [unwired: 9 in]
                }
                frame 2 {
                  n122 = call <vilib>:"sit CONVERT DBL.vi"("Last Row"=w294, "Raw Data"=w295) -> ("Output"=→"Direction R VSP":dbl)  [unwired: 9 in]
                }
                frame 3 {
                  n123 = call <vilib>:"sit CONVERT DBL.vi"("Last Row"=w297, "Raw Data"=w298) -> ("Output"=→"Magnitude Pitch L VSP":dbl)  [unwired: 9 in]
                }
                frame 4 {
                  n124 = call <vilib>:"sit CONVERT DBL.vi"("Last Row"=w300, "Raw Data"=w301) -> ("Output"=→"Magnitude Pitch R VSP":dbl)  [unwired: 9 in]
                }
                frame 5 {
                  n125 = call <vilib>:"sit CONVERT DBL.vi"("Last Row"=w303, "Raw Data"=w304) -> ("Output"=→"Main Battery":dbl)  [unwired: 9 in]
                }
                frame 6 {
                  n126 = call <vilib>:"sit CONVERT DBL.vi"("Last Row"=w306, "Raw Data"=w307) -> ("Output"=→"Main battery half voltage":dbl)  [unwired: 9 in]
                }
                frame 7 {
                  n127 = call <vilib>:"sit CONVERT DBL.vi"("Last Row"=w309, "Raw Data"=w310) -> ("Output"=→"Numeric":dbl)  [unwired: 9 in]
                }
                frame 8 {
                  n128 = call <vilib>:"sit CONVERT DBL.vi"("Last Row"=w312, "Raw Data"=w313) -> ("Output"=→"Numeric 2":dbl)  [unwired: 9 in]
                }
                frame 9 {
                  n129 = call <vilib>:"sit CONVERT WaveformChart.vi"("Timestamps"=w315, "Last Row"=w316, "Raw Data"=w317) -> ("Output"=w314:waveform(dbl)[][])  [unwired: 8 in]
                  n130 = for {
                    tunnel: w314 -> [w318] mode=indexing
                    "Regulation Error East" <- w318
                  }
                }
                frame 10 {
                  n131 = call <vilib>:"sit CONVERT WaveformChart.vi"("Timestamps"=w320, "Last Row"=w321, "Raw Data"=w322) -> ("Output"=w319:waveform(dbl)[][])  [unwired: 8 in]
                  n132 = for {
                    tunnel: w319 -> [w323] mode=indexing
                    "Regulation Error North" <- w323
                  }
                }
                frame 11 {
                  n133 = call <vilib>:"sit CONVERT WaveformChart.vi"("Timestamps"=w325, "Last Row"=w326, "Raw Data"=w327) -> ("Output"=w324:waveform(dbl)[][])  [unwired: 8 in]
                  n134 = for {
                    tunnel: w324 -> [w328] mode=indexing
                    "Regulation Error Yaw" <- w328
                  }
                }
                frame 12 {
                  n135 = call <vilib>:"sit CONVERT DBL.vi"("Last Row"=w330, "Raw Data"=w331) -> ("Output"=→"SIT1":dbl)  [unwired: 9 in]
                }
                frame 13 {
                  n136 = call <vilib>:"sit CONVERT DBL.vi"("Last Row"=w333, "Raw Data"=w334) -> ("Output"=→"SIT1 2":dbl)  [unwired: 9 in]
                }
                frame 14 {
                  n137 = call <vilib>:"sit CONVERT DBL.vi"("Last Row"=w336, "Raw Data"=w337) -> ("Output"=→"SIT1 3":dbl)  [unwired: 9 in]
                }
                frame 15 {
                  n138 = call <vilib>:"sit CONVERT DBL.vi"("Last Row"=w339, "Raw Data"=w340) -> ("Output"=→"SIT1 4":dbl)  [unwired: 9 in]
                }
                frame 16 {
                  n139 = call <vilib>:"sit CONVERT DBL.vi"("Last Row"=w342, "Raw Data"=w343) -> ("Output"=→"SIT1 5":dbl)  [unwired: 9 in]
                }
                frame 17 {
                  n140 = call <vilib>:"sit CONVERT DBL.vi"("Last Row"=w345, "Raw Data"=w346) -> ("Output"=→"SIT1 6":dbl)  [unwired: 9 in]
                }
                frame 18 {
                  n141 = call <vilib>:"sit CONVERT DBL.vi"("Last Row"=w348, "Raw Data"=w349) -> ("Output"=→"SIT1 7":dbl)  [unwired: 9 in]
                }
                frame 19 {
                  n142 = call <vilib>:"sit CONVERT DBL.vi"("Last Row"=w351, "Raw Data"=w352) -> ("Output"=→"SIT1 8":dbl)  [unwired: 9 in]
                }
                frame 20 {
                  n143 = call <vilib>:"sit CONVERT DBL.vi"("Last Row"=w354, "Raw Data"=w355) -> ("Output"=→"SIT1 9":dbl)  [unwired: 9 in]
                }
                frame 21 {
                  n144 = call <vilib>:"sit CONVERT DBL.vi"("Last Row"=w357, "Raw Data"=w358) -> ("Output"=→"Servo Battery":dbl)  [unwired: 9 in]
                }
                frame 22 {
                  n145 = call <vilib>:"sit CONVERT DBL.vi"("Last Row"=w360, "Raw Data"=w361) -> ("Output"=→"Slide BT green":dbl)  [unwired: 9 in]
                }
                frame 23 {
                  n146 = call <vilib>:"sit CONVERT DBL.vi"("Last Row"=w363, "Raw Data"=w364) -> ("Output"=→"Slide BT red":dbl)  [unwired: 9 in]
                }
                frame 24 {
                  n147 = call <vilib>:"sit CONVERT DBL.vi"("Last Row"=w366, "Raw Data"=w367) -> ("Output"=→"Tau_1":dbl)  [unwired: 9 in]
                }
                frame 25 {
                  n148 = call <vilib>:"sit CONVERT DBL.vi"("Last Row"=w369, "Raw Data"=w370) -> ("Output"=→"Tau_2":dbl)  [unwired: 9 in]
                }
                frame 26 {
                  n149 = call <vilib>:"sit CONVERT DBL.vi"("Last Row"=w372, "Raw Data"=w373) -> ("Output"=→"Tau_6":dbl)  [unwired: 9 in]
                }
                frame 27 {
                  n150 = call <vilib>:"sit CONVERT DBL.vi"("Last Row"=w375, "Raw Data"=w376) -> ("Output"=→"Vis E":dbl)  [unwired: 9 in]
                }
                frame 28 {
                  n151 = call <vilib>:"sit CONVERT DBL.vi"("Last Row"=w378, "Raw Data"=w379) -> ("Output"=→"Vis N":dbl)  [unwired: 9 in]
                }
                frame 29 {
                  n152 = call <vilib>:"sit CONVERT DBL.vi"("Last Row"=w381, "Raw Data"=w382) -> ("Output"=→"Vis Pitch":dbl)  [unwired: 9 in]
                }
                frame 30 {
                  n153 = call <vilib>:"sit CONVERT DBL.vi"("Last Row"=w384, "Raw Data"=w385) -> ("Output"=→"Vis Psi":dbl)  [unwired: 9 in]
                }
                frame 31 {
                  n154 = call <vilib>:"sit CONVERT DBL.vi"("Last Row"=w387, "Raw Data"=w388) -> ("Output"=→"Vis Roll":dbl)  [unwired: 9 in]
                }
                frame 32 {
                  n155 = call <vilib>:"sit CONVERT DBL.vi"("Last Row"=w390, "Raw Data"=w391) -> ("Output"=→"Vis X":dbl)  [unwired: 9 in]
                }
                frame 33 {
                  n156 = call <vilib>:"sit CONVERT DBL.vi"("Last Row"=w393, "Raw Data"=w394) -> ("Output"=→"Vis Y":dbl)  [unwired: 9 in]
                }
                frame 34 {
                  n157 = call <vilib>:"sit CONVERT DBL.vi"("Last Row"=w396, "Raw Data"=w397) -> ("Output"=→"Vis Yaw":dbl)  [unwired: 9 in]
                }
                frame 35 {
                  n158 = call <vilib>:"sit CONVERT DBL.vi"("Last Row"=w399, "Raw Data"=w400) -> ("Output"=→"Vis Z":dbl)  [unwired: 9 in]
                }
                frame 36 {
                  n159 = call <vilib>:"sit CONVERT Boolean.vi"("Last Row"=w402, "Raw Data"=w403) -> ("Output"=→"X button":bool)  [unwired: 9 in]
                }
                frame 37 {
                  n160 = call <vilib>:"sit CONVERT DBL.vi"("Last Row"=w405, "Raw Data"=w406) -> ("Output"=→"port vsp r":dbl)  [unwired: 9 in]
                }
                frame 38 {
                  n161 = call <vilib>:"sit CONVERT DBL.vi"("Last Row"=w408, "Raw Data"=w409) -> ("Output"=→"stbd vsp r":dbl)  [unwired: 9 in]
                }
                frame 39 {
                  n162 = call <vilib>:"sit CONVERT DBL.vi"("Last Row"=w411, "Raw Data"=w412) -> ("Output"=→"u1":dbl)  [unwired: 9 in]
                }
                frame 40 {
                  n163 = call <vilib>:"sit CONVERT DBL.vi"("Last Row"=w414, "Raw Data"=w415) -> ("Output"=→"u2":dbl)  [unwired: 9 in]
                }
                frame 41 {
                  n164 = call <vilib>:"sit CONVERT DBL.vi"("Last Row"=w417, "Raw Data"=w418) -> ("Output"=→"u3":dbl)  [unwired: 9 in]
                }
                frame 42 {
                  n165 = call <vilib>:"sit CONVERT DBL.vi"("Last Row"=w420, "Raw Data"=w421) -> ("Output"=→"u4":dbl)  [unwired: 9 in]
                }
                frame 43 {
                  n166 = call <vilib>:"sit CONVERT DBL.vi"("Last Row"=w423, "Raw Data"=w424) -> ("Output"=→"u5":dbl)  [unwired: 9 in]
                }
              }
            }
          }
        }
        n167 = call <vilib>:"sit Check to Stop Client.vi"("error in (no error)"=w264) -> ("error out"=w265:errorcluster, "Stop?"=w263:bool)  [unwired: 2 in, 7 out]
        n168 = Wait (ms)(milliseconds to wait=u32 50) -> ()  [unwired: 1 out]
      }
      n169 = local write "SIT_Meta_Info"(w170) -> ()
      n170 = call <vilib>:"sit Merge SIT Client Errors.vi"("Bottom Loop Error"=w166, "Top Loop Error"=w164) -> ("Resulting Error"=w165:errorcluster)  [unwired: 9 out]
    }
    frame Error {
      # "User canceled target selection (or an error occurred on Init)...don't run the client"
      n171 = local write "SIT_Meta_Info"(w425) -> ()
    }
  }
  n172 = call-poly <vilib>:"Close Input Device.vi"("error in (no error)"=w55, "device ID"=w56) -> ("error out"=w48:errorcluster)  [unwired: 8 out]
  n173 = local write "SIT_stopVI"(w65) -> ()
  n174 = call <vilib>:"sit Clear Client.vi"("error in (no error)"=w71, "SIT Client Op Refs"=w67) -> ("error out"=w68:errorcluster)  [unwired: 9 out]
  n175 = call <vilib>:"sit Check to Stop Client.vi"("Reset Stop?"=TRUE ("Clear Item?"), "error in (no error)"=w68) -> ("error out"=w60:errorcluster)  [unwired: 1 in, 8 out]
  n176 = call <vilib>:"sit Check Run-Time System.vi"("error in"=w60) -> ("Run Time System?"=w59:bool)  [unwired: 10 out]
  n177 = Quit LabVIEW(quit? (T)=w59) -> ()
  n178 = call <vilib>:"General Error Handler.vi"("error in (no error)"=w48) -> ()  [unwired: 1 in, 14 out]
  n179 = call <vilib>:"Load VRML File.vi"("Path"=path "C:/Documents and Settings/mcl/My Documents/LabView/CSEnterpriseI/boat/target2.wrl") -> ("Scene:Read Scene File"=w6:refnum<vi>)  [unwired: 9 in, 1 out]
  n180 = call <vilib>:"Load VRML File.vi"("Path"=path "C:/Documents and Settings/mcl/My Documents/LabView/CSEnterpriseI/boat/3dsboat55.wrl") -> ("Scene:Read Scene File"=w29:refnum<vi>)  [unwired: 9 in, 1 out]
  n181 = call <vilib>:"Create Object.vi"() -> ("Scene:New Object"=w7:refnum<vi>)  [unwired: 10 in, 1 out]
  n182 = invoke on="3D Picture" class="SceneGraphDisp (strict)" method="Setup Camera"("Camera Position"=cluster{"X":sgl, "Y":sgl, "Z":sgl} {"X"=-3.0, "Y"=3.0, "Z"=0.0}, "Target"=cluster{"X":sgl, "Y":sgl, "Z":sgl} {"X"=0.0, "Y"=0.0, "Z"=0.0} ("Camera Position"), "Up Direction"=cluster{"X":sgl, "Y":sgl, "Z":sgl} {"X"=1.0, "Y"=0.0, "Z"=0.0} ("Camera Position")) -> ()  [unwired: 3 in, 6 out]
  n183 = call <vilib>:"Load VRML File.vi"("Path"=path "C:/Documents and Settings/mcl/My Documents/LabView/CSEnterpriseI/boat/3dsboatv2_yellow.wrl") -> ("Scene:Read Scene File"=w36:refnum<vi>)  [unwired: 9 in, 1 out]
  n184 = call <vilib>:"Create Object.vi"() -> ("Scene:New Object"=w30:refnum<vi>)  [unwired: 10 in, 1 out]
  n185 = call <vilib>:"Create Object.vi"() -> ("Scene:New Object"=w41:refnum<vi>)  [unwired: 10 in, 1 out]
  n186 = call <vilib>:"Create Box.vi"("Color"=T11 {"Red"=0.0, "Green"=0.0, "Blue"=1.0, "Alpha"=1.0}, "Length Z"=sgl 6.5 ("Red"), "Length Y"=sgl 0.001 ("Red"), "Length X"=sgl 20.0 ("Red")) -> ("New Box Refnum"=w40:refnum<vi>)  [unwired: 6 in, 1 out]
  n187 = call <vilib>:"Create Object.vi"() -> ("Scene:New Object"=w37:refnum<vi>)  [unwired: 10 in, 1 out]
  n188 = invoke class="SceneObject" method="Object.Add Object"(reference=w7, "Child"=w6) -> (reference out=w3:refnum<vi>, "Child"=w2:refnum<vi>)  [unwired: 2 in, 2 out]
  n189 = invoke class="SceneObject" method="Object.Add Object"(reference=w30, "Child"=w29) -> (reference out=w26:refnum<vi>, "Child"=w22:refnum<vi>)  [unwired: 2 in, 2 out]
  n190 = invoke class="SceneObject" method="Set Geometry"(reference=w41, "Param 0"=w40) -> (reference out=w32:refnum<vi>)  [unwired: 2 in, 3 out]
  n191 = invoke class="SceneObject" method="Object.Add Object"(reference=w37, "Child"=w36) -> (reference out=w28:refnum<vi>, "Child"=w23:refnum<vi>)  [unwired: 2 in, 2 out]
  n192 = invoke class="SceneObject" method="Object.Add Object"(reference=w28, "Child"=w26) -> (reference out=w27:refnum<vi>)  [unwired: 2 in, 3 out]
  n193 = call <vilib>:"Set Scale.vi"("Scale"=cluster{"X":sgl, "Y":sgl, "Z":sgl} {"X"=0.001, "Y"=0.001, "Z"=0.001} ("Camera Position"), "Scene Object"=w22) -> ("Scaled Object"=w1:refnum<vi>)  [unwired: 8 in, 1 out]
  n194 = invoke class="SceneObject" method="Object.Add Object"(reference=w27, "Child"=w32) -> (reference out=w5:refnum<vi>)  [unwired: 2 in, 3 out]
  n195 = property on="3D Picture" class="SceneGraphDisp (strict)"("Background Color"=cluster{"X":sgl, "Y":sgl, "Z":sgl, "Z 2":sgl} {"X"=1.0, "Y"=1.0, "Z"=1.0, "Z 2"=1.0} ("Camera Position")) -> ()  [unwired: 2 in, 2 out]
  n196 = invoke class="SceneObject" method="Object.Add Object"(reference=w5, "Child"=w3) -> (reference out=w4:refnum<vi>)  [unwired: 2 in, 3 out]
  n197 = call <vilib>:"Create Box.vi"("Color"=T11 {"Red"=1.0, "Green"=0.0, "Blue"=0.0, "Alpha"=1.0}, "Length Z"=sgl 0.1 ("Red"), "Length Y"=sgl 0.1 ("Red"), "Length X"=sgl 3.0 ("Red")) -> ("New Box Refnum"=w21:refnum<vi>)  [unwired: 6 in, 1 out]
  n198 = call <vilib>:"Create Object.vi"() -> ("Scene:New Object"=w16:refnum<vi>)  [unwired: 10 in, 1 out]
  n199 = invoke class="SceneObject" method="Set Geometry"(reference=w16, "Param 0"=w21) -> ()  [unwired: 2 in, 4 out]
  n200 = call <vilib>:"Create Box.vi"("Color"=T11 {"Red"=0.0, "Green"=1.0, "Blue"=0.0, "Alpha"=1.0}, "Length Z"=sgl 0.1 ("Red"), "Length Y"=sgl 3.0 ("Red"), "Length X"=sgl 0.1 ("Red")) -> ("New Box Refnum"=w15:refnum<vi>)  [unwired: 6 in, 1 out]
  n201 = call <vilib>:"Create Object.vi"() -> ("Scene:New Object"=w11:refnum<vi>)  [unwired: 10 in, 1 out]
  n202 = invoke class="SceneObject" method="Set Geometry"(reference=w11, "Param 0"=w15) -> ()  [unwired: 2 in, 4 out]
  n203 = call <vilib>:"Set Scale.vi"("Scale"=cluster{"X":sgl, "Y":sgl, "Z":sgl} {"X"=0.001, "Y"=0.001, "Z"=0.001} ("Camera Position"), "Scene Object"=w23) -> ("Scaled Object"=w9:refnum<vi>)  [unwired: 8 in, 1 out]
  n204 = while {
    tunnel: w4 -> [w437]
    tunnel: w9 -> [w435]
    tunnel: w2 -> [w432]
    tunnel: w1 -> [w429]
    stop <- w434 stop-if-true
    n205 = flat-sequence {
      tunnel: w437 -> [w487]
      tunnel: [w487] -> w436
      tunnel: w435 -> [w486]
      tunnel: w432 -> [w481]
      tunnel: w429 -> [w464]
      tunnel: w436 -> [w497]
      tunnel: [w497] -> w433
      frame #0 {
        (unwired) sgl 0.0 ("Red")
        n206 = Boolean To (0,1)(Boolean="OK Button") -> (0, 1=w453:i16)
        n207 = Boolean To (0,1)(Boolean="USE cse1 setpoint") -> (0, 1=w448:i16)
        n208 = Multiply(x=w448, y=2) -> (x*y=w449:i32)
        n209 = Add(x=w449, y=w453) -> (x+y=w454:i32)
        n210 = Not(x="Show HIL") -> (.not. x?=w443:bool)
        n211 = Not(x="Show CSEI") -> (.not. x?=w438:bool)
        n212 = property on="Vis E" class="DigNum (strict)"() -> ("Value"=w474:dbl)  [unwired: 2 in, 2 out]
        n213 = property on="Vis N" class="DigNum (strict)"() -> ("Value"=w476:dbl)  [unwired: 2 in, 2 out]
        n214 = property on="Vis X" class="DigNum (strict)"() -> ("Value"=w452:dbl)  [unwired: 2 in, 2 out]
        n215 = property on="Vis Y" class="DigNum (strict)"() -> ("Value"=w451:dbl)  [unwired: 2 in, 2 out]
        n216 = property on="Vis Z" class="DigNum (strict)" props=["Value"]() -> ()  [unwired: 2 in, 3 out]
        n217 = Boolean To (0,1)(Boolean=w438) -> (0, 1=w446:i16)
        n218 = Boolean To (0,1)(Boolean=w443) -> (0, 1=w441:i16)
        n219 = Multiply(x=w441, y=-1) -> (x*y=w440:i32)
        n220 = Multiply(x=w451, y=1) -> (x*y=w460:dbl)
        n221 = Multiply(x=w446, y=-1) -> (x*y=w458:i32)
        n222 = Multiply(x=w452, y=1) -> (x*y=w462:dbl)
        n223 = Bundle("Value"=w476, w440, "Value"=w474) -> (w485:cluster{"Value":dbl, i32, "Value":dbl})  [unwired: 1 in]
        n224 = property on="Vis Psi" class="DigNum (strict)"() -> ("Value"=w475:dbl)  [unwired: 2 in, 2 out]
        n225 = Bundle(w462, w458, w460) -> (w465:cluster{dbl, i32, dbl})  [unwired: 1 in]
        n226 = call <vilib>:"Set Translation.vi"("Translation"=w465, "Scene Object"=w464) -> ("Translated Object"=w467:refnum<vi>)  [unwired: 8 in, 1 out]
        n227 = property on="Vis Yaw" class="DigNum (strict)"() -> ("Value"=w450:dbl)  [unwired: 2 in, 2 out]
        n228 = case shown="2" w454 {
          tunnel: w476 -> [_ w493 _]
          tunnel: "eta_d_N" -> [w488 _ _]
          tunnel: "eta_d_Psi" -> [w489 _ _]
          tunnel: w475 -> [_ w491 _]
          tunnel: "eta_d_E" -> [w490 _ _]
          tunnel: w474 -> [_ w492 _]
          tunnel: [w488 w493 w496] -> w471
          tunnel: [w490 w492 w495] -> w473
          tunnel: [w489 w491 w494] -> w472
          tunnel: w452 -> [_ _ w496]
          tunnel: w451 -> [_ _ w495]
          tunnel: w450 -> [_ _ w494]
          frame 0, Default {
          }
          frame 1 {
          }
          frame 2 {
          }
        }
        n229 = property on="eta_d_N" class="DigNum (strict)"("Val(Sgnl)"=w471) -> ()  [unwired: 2 in, 2 out]
        n230 = Bundle("Value"=w471, "Red"=sgl 0.0, "eta_d_E"="eta_d_E") -> (w480:cluster{"Value":dbl, "Red":sgl, "eta_d_E":dbl})  [unwired: 1 in]
        n231 = Negate(x="eta_d_Psi") -> (-x=w477:dbl)
        n232 = call <vilib>:"Set Translation.vi"("Translation"=w485, "Scene Object"=w486) -> ("Translated Object"=w483:refnum<vi>)  [unwired: 8 in, 1 out]
        n233 = property on="eta_d_E" class="DigNum (strict)"("Val(Sgnl)"=w473) -> ()  [unwired: 2 in, 2 out]
        n234 = call <vilib>:"Set Translation.vi"("Translation"=w480, "Scene Object"=w481) -> ("Translated Object"=w479:refnum<vi>)  [unwired: 8 in, 1 out]
        n235 = property on="eta_d_Psi" class="DigNum (strict)"("Val(Sgnl)"=w472) -> ()  [unwired: 2 in, 2 out]
        n236 = Negate(x=w450) -> (-x=w457:dbl)
        n237 = Negate(x=w475) -> (-x=w482:dbl)
        n238 = call <vilib>:"Set Rotation.vi"("Angle"=w482, "Axis"=cluster{"X":sgl, "Y":sgl, "Z":sgl} {"X"=0.0, "Y"=1.0, "Z"=0.0} ("Camera Position"), "Scene Object"=w483) -> ()  [unwired: 7 in, 2 out]
        n239 = call <vilib>:"Set Rotation.vi"("Angle"=w457, "Axis"=cluster{"X":sgl, "Y":sgl, "Z":sgl} {"X"=0.0, "Y"=1.0, "Z"=0.0} ("Camera Position"), "Scene Object"=w467) -> ()  [unwired: 7 in, 2 out]
        n240 = property on="Vis Roll" class="DigNum (strict)" props=["Value"]() -> ()  [unwired: 2 in, 3 out]
        n241 = call <vilib>:"Set Rotation.vi"("Angle"=w477, "Axis"=cluster{"X":sgl, "Y":sgl, "Z":sgl} {"X"=0.0, "Y"=1.0, "Z"=0.0} ("Camera Position"), "Scene Object"=w479) -> ()  [unwired: 7 in, 2 out]
        n242 = property on="Vis Pitch" class="DigNum (strict)" props=["Value"]() -> ()  [unwired: 2 in, 3 out]
      }
      frame #1 {
        n243 = Wait (ms)(milliseconds to wait=u32 50) -> ()  [unwired: 1 out]
      }
    }
    n244 = Boolean To (0,1)(Boolean="HIL -> CSE1") -> (0, 1=w430:i16)
    n245 = Boolean To (0,1)(Boolean="Resed DP Int.") -> (0, 1=w427:i16)
    n246 = property on="Reset States" class="DigNum (strict)"("Val(Sgnl)"=w430) -> ()  [unwired: 2 in, 2 out]
    n247 = property on="Reset dp" class="DigNum (strict)"("Val(Sgnl)"=w427) -> ()  [unwired: 2 in, 2 out]
    n248 = property on="SIT_stopVI" class="Bool (strict)"() -> ("Value"=w434:bool)  [unwired: 2 in, 2 out]
    "3D Picture" <- w433
  }
